vi "GetQueueNameByLogName.vi"(8 "error in (no error)":errorcluster, 11 "LogName":string) -> (0 "error out":errorcluster, 3 "QueueName":string)   [LabVIEW 2016, in "Log4Lv.lvlib"]
doc: "Use this template to build a VI to use as a subVI."
uses:
  Log4Lv.lvlib
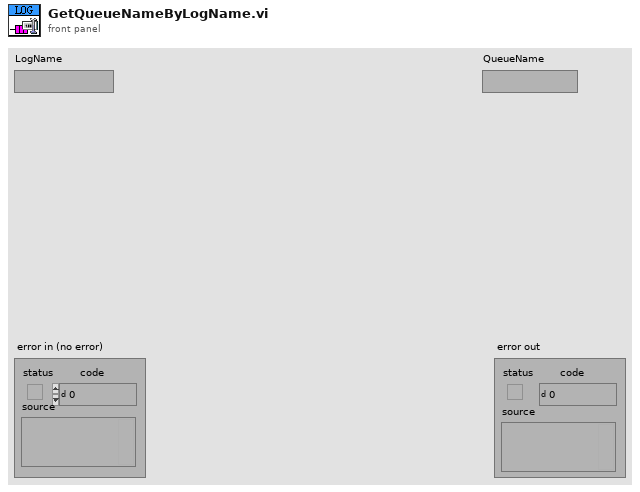
[diagram p1: front panel]
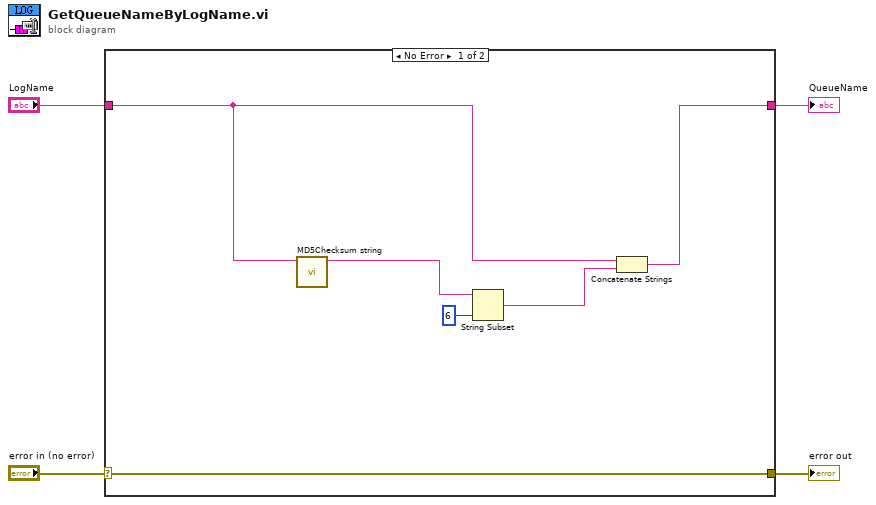
[diagram p0: block diagram]
diagram:
  n1 = case shown="No Error" "error in (no error)" {
    selector: "error in (no error)" -> [w10 w12]
    tunnel: [w10 w12] -> w3
    tunnel: "LogName" -> [w9 w11]
    tunnel: [w8 w11] -> w1
    frame No Error {
      n2 = call <vilib>:"MD5Checksum string.vi"("Message String"=w9) -> ("MD5 message-digest"=w6:string)  [unwired: 10 in]
      n3 = String Subset(string=w6, length (rest)=6 ("length (rest)")) -> (substring=w5:string)  [unwired: 1 in]
      n4 = Concatenate Strings(w9, w5) -> (w8:string)
    }
    frame Error {
    }
  }
  "error out" <- w3
  "QueueName" <- w1
